vi "op_rel_v2.vi"() -> ()   [LabVIEW 2009]
panel:
  out "L9":bool
  out "L8":bool
  in  "Knob":u8(knob) scale=0.0..9.0
  out "L0":bool
  out "L1":bool
  out "L2":bool
  out "L3":bool
  out "L4":bool
  out "L5":bool
  out "L6":bool
  out "L7":bool
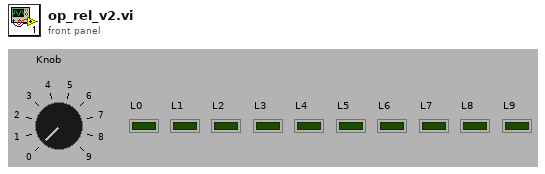
[diagram p1: front panel]
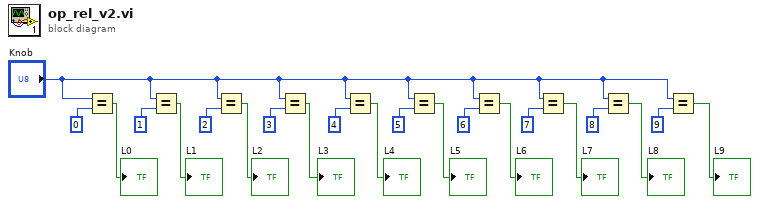
[diagram p0: block diagram]
diagram:
  n1 = Equal?(x="Knob", y=0) -> (x = y?=→"L0":bool)
  n2 = Equal?(x="Knob", y=1) -> (x = y?=→"L1":bool)
  n3 = Equal?(x="Knob", y=2) -> (x = y?=→"L2":bool)
  n4 = Equal?(x="Knob", y=3) -> (x = y?=→"L3":bool)
  n5 = Equal?(x="Knob", y=4) -> (x = y?=→"L4":bool)
  n6 = Equal?(x="Knob", y=5) -> (x = y?=→"L5":bool)
  n7 = Equal?(x="Knob", y=6) -> (x = y?=→"L6":bool)
  n8 = Equal?(x="Knob", y=7) -> (x = y?=→"L7":bool)
  n9 = Equal?(x="Knob", y=8) -> (x = y?=→"L8":bool)
  n10 = Equal?(x="Knob", y=9) -> (x = y?=→"L9":bool)
